vi "OEE_SCREEN_2_worst_pace_into_cluster.vi"(6 "SCREEN_2":T1={"header_part_no"="-", "header_customer"="-", "performance_percentage"="-", "performance_target"="-", "performance_actual"="-", "performance_header"="PERFORMANCE", "performance_header_target"="TARGET", "performance_header_actual"="ACTUAL"}, 11 "pace_from_worst":i32[][](array[numeric])) -> (4 "SCREEN_2":T1={"header_part_no"="-", "header_customer"="-", "performance_percentage"="-", "performance_target"="-", "performance_actual"="-", "performance_header"="PERFORMANCE", "performance_header_target"="TARGET", "performance_header_actual"="ACTUAL"})   [LabVIEW 2019]
uses:
  typedef/SCREEN_2.ctl
panel:
  # "Performance Data Output Board #2"
  # "Performance Data Output Board #2"
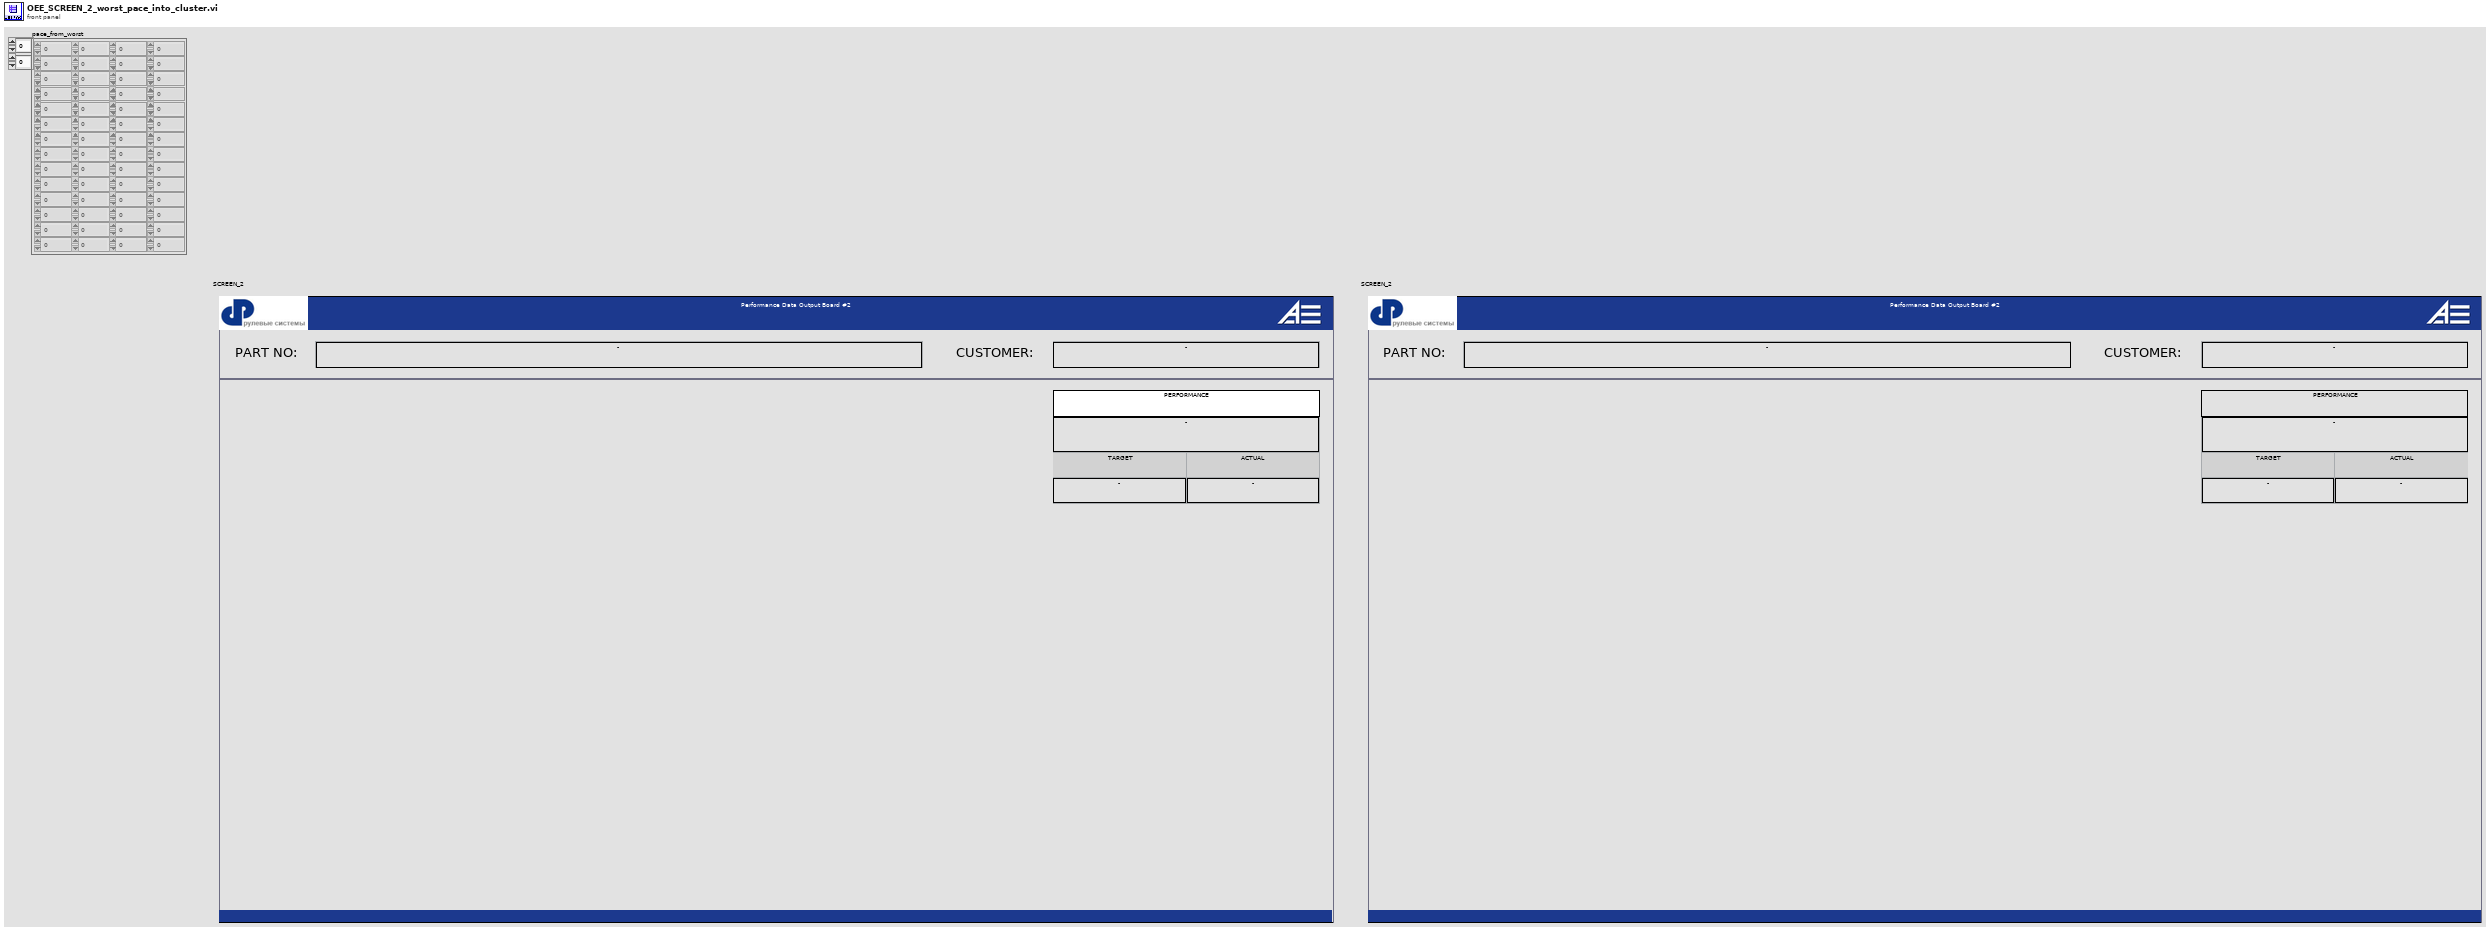
[diagram p1: front panel]
types:
  T1 = typedef "SCREEN_2.ctl" = cluster{"header_part_no":string, "header_customer":string, "performance_percentage":string, "performance_target":string, "performance_actual":string, "performance_header":string, "performance_header_target":string, "performance_header_actual":string}
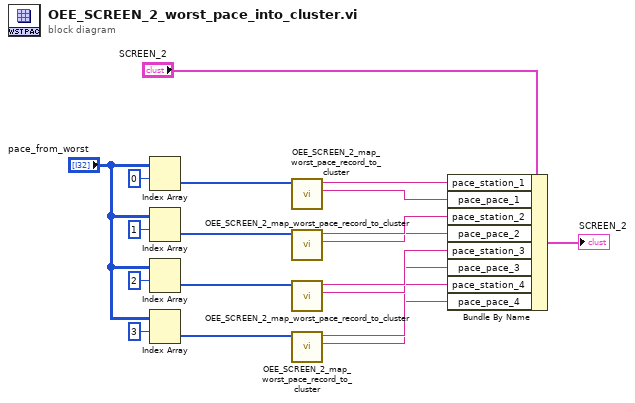
[diagram p0: block diagram]
diagram:
  n1 = Index Array(array="pace_from_worst", index (row)=0) -> (element=w12:i32[])  [unwired: 1 in]
  n2 = Index Array(array="pace_from_worst", index (row)=1) -> (element=w7:i32[])  [unwired: 1 in]
  n3 = Index Array(array="pace_from_worst", index (row)=2) -> (element=w8:i32[])  [unwired: 1 in]
  n4 = Index Array(array="pace_from_worst", index (row)=3) -> (element=w9:i32[])  [unwired: 1 in]
  n5 = call "OEE_SCREEN_2_map_worst_pace_record_to_cluster.vi"("pace_record"=w12) -> ("pace"=w10:string, "station"=w11:string)  [unwired: 9 in]
  n6 = call "OEE_SCREEN_2_map_worst_pace_record_to_cluster.vi"("pace_record"=w7) -> ("pace"=w5:string, "station"=w6:string)  [unwired: 9 in]
  n7 = call "OEE_SCREEN_2_map_worst_pace_record_to_cluster.vi"("pace_record"=w8) -> ("pace"=w3:string, "station"=w4:string)  [unwired: 9 in]
  n8 = call "OEE_SCREEN_2_map_worst_pace_record_to_cluster.vi"("pace_record"=w9) -> ("pace"=w1:string, "station"=w2:string)  [unwired: 9 in]
  n9 = Bundle By Name(cluster="SCREEN_2", "pace_station_1"=w11, "pace_pace_1"=w10, "pace_station_2"=w6, "pace_pace_2"=w5, "pace_station_3"=w4, "pace_pace_3"=w3, "pace_station_4"=w2, "pace_pace_4"=w1) -> (→"SCREEN_2":T1)
